vi "Configure Noise Level.vi"(8 "error in":errorcluster, 10 "level":dbl, 11 "lia host in":refnum<class "LIA Host Interface FPGA.lvclass">) -> (0 "error out":errorcluster, 3 "lia host out":refnum<class "LIA Host Interface FPGA.lvclass">)   [LabVIEW 2018, in "LIA Host Interface FPGA.lvclass"]
uses:
  LIA Host Interface FPGA.lvclass
  Properties/FpgaSession_GET.vi
  host/Lock-In Amplifier Example Host.lvlib
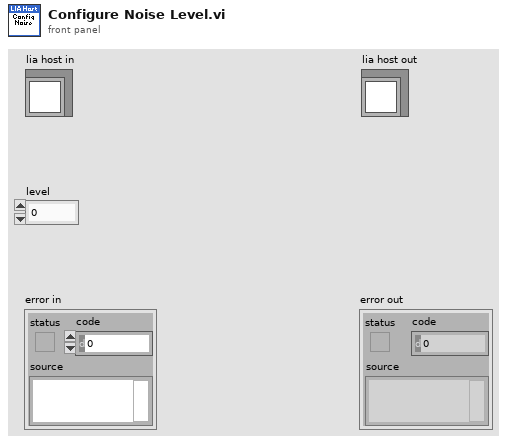
[diagram p1: front panel]
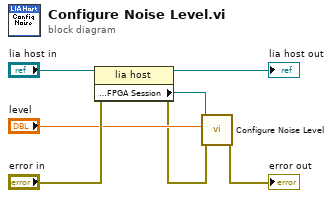
[diagram p0: block diagram]
diagram:
  n1 = property class="lia host"(reference="lia host in", error in="error in") -> (reference out=→"lia host out":refnum<class "LIA Host Interface FPGA.lvclass">, error out=w2:errorcluster, "Properties:FPGA Session"=w4:refnum<k20>)
  n2 = call "Configure Noise Level.vi"("error in"=w2, "level"="level", "fpga session in"=w4) -> ("error out"=→"error out":errorcluster)  [unwired: 7 in, 1 out]
